vi "PalmSense Get Current Range.vi"() -> (1 "Start Current Range":i32, 2 "Max Current Range":i32, 3 "Min Current Range":i32)   [LabVIEW 2020, in "PalmSens.lvlib"]
uses:
  PalmSens.lvlib
  support/PCT FGV CMD.ctl
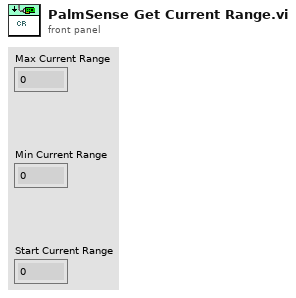
[diagram p1: front panel]
types:
  T1 = typedef "PCT FGV CMD.ctl" = enum16{"INIT", "GET", "SET"}
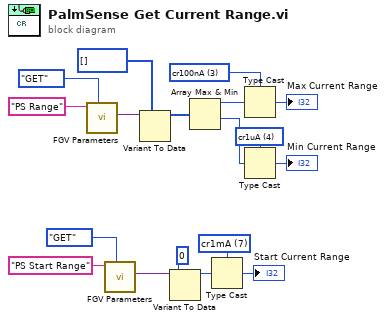
[diagram p0: block diagram]
diagram:
  w15 = 7 items=["cr100pA"=0, "cr1nA"=1, "cr10nA"=2, "cr100nA"=3, "cr1uA"=4, "cr10uA"=5, "cr100uA"=6, "cr1mA"=7, "cr10mA"=8, "cr100mA"=9, "cr2uA"=10, "cr4uA"=11, "cr8uA"=12, "cr16uA"=13, "cr32uA"=14, "cr125uA"=17, "cr250uA"=18, "cr500uA"=19, "cr5mA"=20, "cr6uA"=21, "cr13uA"=22, "cr25uA"=23, "cr50uA"=24, "cr200uA"=25, "cr63uA"=26] ("cr")
  w12 = 4 items=["cr100pA"=0, "cr1nA"=1, "cr10nA"=2, "cr100nA"=3, "cr1uA"=4, "cr10uA"=5, "cr100uA"=6, "cr1mA"=7, "cr10mA"=8, "cr100mA"=9, "cr2uA"=10, "cr4uA"=11, "cr8uA"=12, "cr16uA"=13, "cr32uA"=14, "cr125uA"=17, "cr250uA"=18, "cr500uA"=19, "cr5mA"=20, "cr6uA"=21, "cr13uA"=22, "cr25uA"=23, "cr50uA"=24, "cr200uA"=25, "cr63uA"=26] ("cr")
  w11 = 3 items=["cr100pA"=0, "cr1nA"=1, "cr10nA"=2, "cr100nA"=3, "cr1uA"=4, "cr10uA"=5, "cr100uA"=6, "cr1mA"=7, "cr10mA"=8, "cr100mA"=9, "cr2uA"=10, "cr4uA"=11, "cr8uA"=12, "cr16uA"=13, "cr32uA"=14, "cr125uA"=17, "cr250uA"=18, "cr500uA"=19, "cr5mA"=20, "cr6uA"=21, "cr13uA"=22, "cr25uA"=23, "cr50uA"=24, "cr200uA"=25, "cr63uA"=26] ("cr")
  n1 = call "FGV Parameters.vi"("CMD"=PCT_FGV_CMD."GET", "Key"="PS Range") -> ("output"=w7:variant)  [unwired: 7 in, 2 out]
  n2 = call "FGV Parameters.vi"("CMD"=PCT_FGV_CMD."GET", "Key"="PS Start Range") -> ("output"=w6:variant)  [unwired: 7 in, 2 out]
  n3 = Variant To Data(type=i32[] [] ("NewVal"), Variant=w7) -> (data=w9:i32[])  [unwired: 1 in, 1 out]
  n4 = Variant To Data(type=0 ("Row"), Variant=w6) -> (data=w14:i32)  [unwired: 1 in, 1 out]
  n5 = Array Max & Min(array=w9) -> (max value=w10:i32, min value=w13:i32)  [unwired: 2 out]
  n6 = Type Cast(type=w15, x=w14) -> (*(type *) &x=→"Start Current Range":i32)
  n7 = Type Cast(type=w11, x=w10) -> (*(type *) &x=→"Max Current Range":i32)
  n8 = Type Cast(type=w12, x=w13) -> (*(type *) &x=→"Min Current Range":i32)
